vi "init_DAC_700b_ai_chans.vi"(10 "Sample Rate":dbl) -> (0 "error out":errorcluster, 1 "Number Chans":dbl, 3 "Refnum out":refnum<k21>)   [LabVIEW 2015]
uses:
  <vilib>/DAQmx/create/channels.llb/DAQmx Create Channel (AI-Voltage-Basic).vi
  <vilib>/DAQmx/configure/timing.llb/DAQmx Timing (Sample Clock).vi
  <resource>/objmgr/daqmx.rc
panel:
  out "Actual Sample Rate Dev1":dbl=1000.0 format="%0.2f"
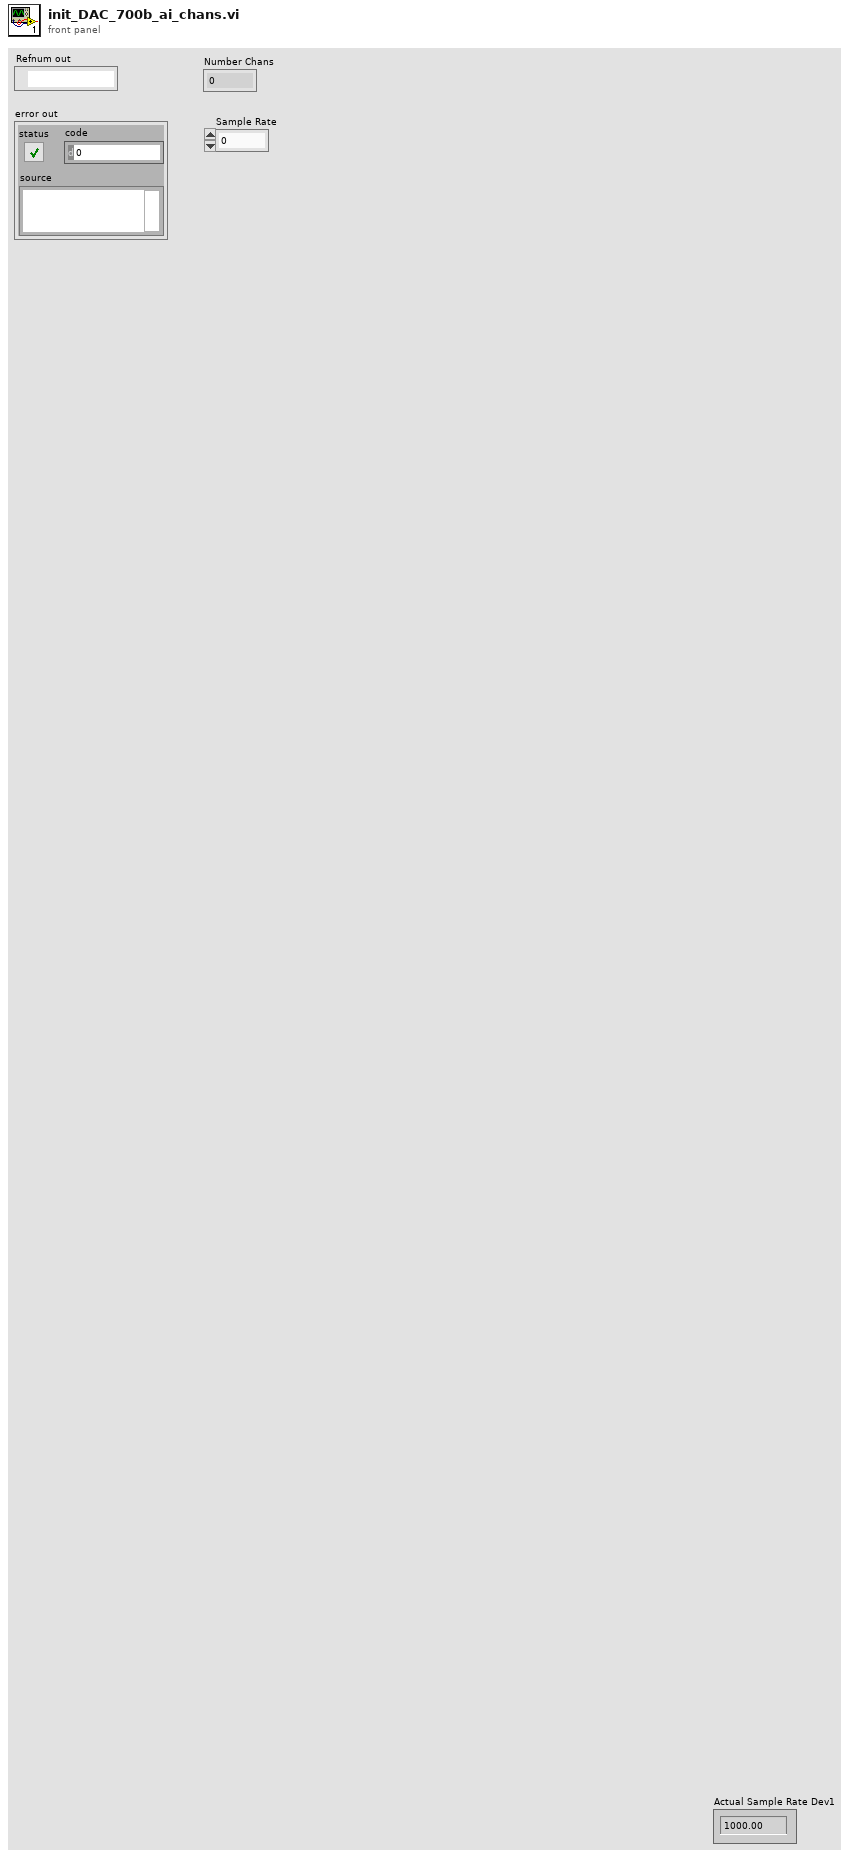
[diagram p1: front panel]
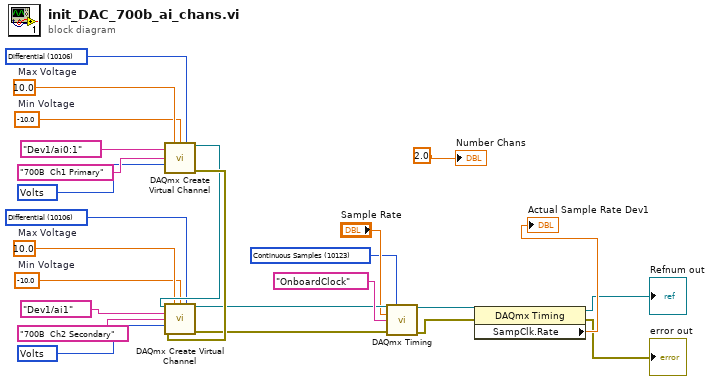
[diagram p0: block diagram]
diagram:
  w1 = 10123 items=["Finite Samples"=10178, "Continuous Samples"=10123] ("sample mode")
  w19 = 10348 items=["Volts"=10348, "From Custom Scale"=10065] ("units")
  w18 = 10106 items=["default"=-1, "RSE"=10083, "NRSE"=10078, "Differential"=10106, "Pseudodifferential"=12529] ("input terminal configuration")
  w16 = -10.0  # Min Voltage
  w17 = 10.0  # Max Voltage
  w15 = 10348 items=["Volts"=10348, "From Custom Scale"=10065] ("units")
  w14 = 10106 items=["default"=-1, "RSE"=10083, "NRSE"=10078, "Differential"=10106, "Pseudodifferential"=12529] ("input terminal configuration")
  w12 = -10.0  # Min Voltage
  w13 = 10.0  # Max Voltage
  n1 = call-poly <vilib>:"DAQmx Create Virtual Channel.vi"("maximum value"=w13, "minimum value"=w12, "input terminal configuration"=w14, "physical channels"=tag "Dev1/ai0:1" ("DAQmx Physical Channel"), "name to assign"="700B  Ch1 Primary", "units"=w15) -> ("task out"=w21:refnum<k21>, "error out"=w22:errorcluster)  [unwired: 8 in]
  n2 = call-poly <vilib>:"DAQmx Create Virtual Channel.vi"("task in"=w21, "maximum value"=w17, "minimum value"=w16, "input terminal configuration"=w18, "physical channels"=tag "Dev1/ai1" ("DAQmx Physical Channel"), "name to assign"="700B  Ch2 Secondary", "units"=w19, "error in"=w22) -> ("task out"=w6:refnum<k21>, "error out"=w5:errorcluster)  [unwired: 6 in]
  n3 = call-poly <vilib>:"DAQmx Timing.vi"("task/channels in"=w6, "sample mode"=w1, "rate"="Sample Rate", "source"=tag "OnboardClock" ("Sample Clock Source"), "error in"=w5) -> ("task out"=w10:refnum<k21>, "error out"=w9:errorcluster)  [unwired: 9 in]
  n4 = property class="DAQmx Timing"(reference=w10, error in=w9) -> (reference out=→"Refnum out":refnum<k21>, error out=→"error out":errorcluster, "SampClk.Rate"=→"Actual Sample Rate Dev1":dbl)
  "Number Chans" <- 2.0 ("Number Chans")
